vi "PicoScope6000Stop.vi"(8 "error in (no error)":errorcluster, 11 "handle":i16) -> (0 "error out":errorcluster, 3 "handle out":i16)   [LabVIEW 2009]
doc: "This closes the oscilloscope and should be called before exiting an application."
uses:
  ps6000.dll
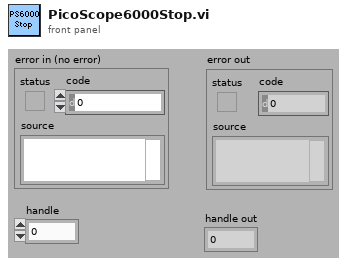
[diagram p1: front panel]
types:
  T1 = cluster{"status":bool, "code":u32, "source":string}
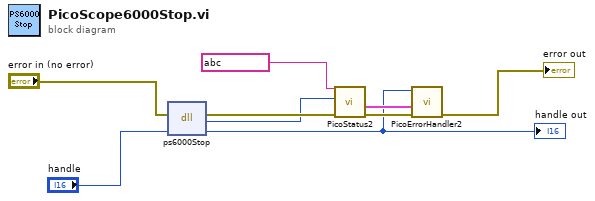
[diagram p0: block diagram]
diagram:
  n1 = dll-call lib="PS6000.dll" fn="ps6000Stop" ("ps3000.dll:_ps3000_open_unit@0")(error in="error in (no error)", "handle"="handle") -> (error out=w5:errorcluster, "PICO_STATUS"=w4:u32, "handle"=w3:i16)  [unwired: 2 in, 1 out]
  "handle out" <- w3
  n2 = call "PicoStatus2.vi"("PICO source"=string ? ("source"), "Error in"=w5, "PICO STATUS"=w4) -> ("error out"=w8:errorcluster, "PICO_STATUS out"=w7:T1)  [unwired: 5 in]
  n3 = call "PicoErrorHandler2.vi"("error in (no error)"=w8, "PICO_STATUS in"=w7, "handle In"=w3) -> ("error out"=→"error out":errorcluster)  [unwired: 8 in]
